vi "Write UI elements.vi"(10 "UI elements":T1, 11 "Controller in":refnum<class "Controller.lvclass">) -> (3 "Controller out":refnum<class "Controller.lvclass">)   [LabVIEW 2011, in "Controller.lvclass"]
uses:
  Controller.lvclass
  Controls/UI Elements.ctl
  Controller.lvclass/Controller.ctl
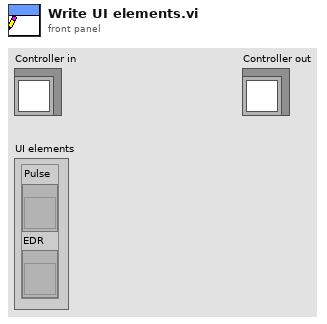
[diagram p1: front panel]
types:
  T1 = typedef "Controller.lvclass/UI Elements.ctl" = cluster{"Pulse":refnum<vi>, "EDR":refnum<vi>}
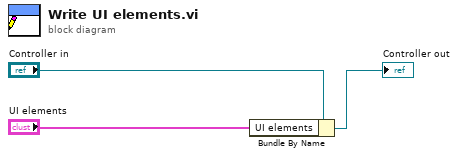
[diagram p0: block diagram]
diagram:
  n1 = Bundle By Name(cluster="Controller in", "UI elements"="UI elements") -> (→"Controller out":refnum<class "Controller.lvclass">)
